vi "Get-pulse-durations.vi"(8 "error in (no error)":errorcluster) -> (0 "error out":errorcluster, 2 "Formatted contents":string)   [LabVIEW 2013, in "MaterialCharacterization.lvlib" / "MC-SM1000.lvclass"]
uses:
  MC-SM1000.lvclass
panel:
  in  "Raw signal":u8[](array[numeric])
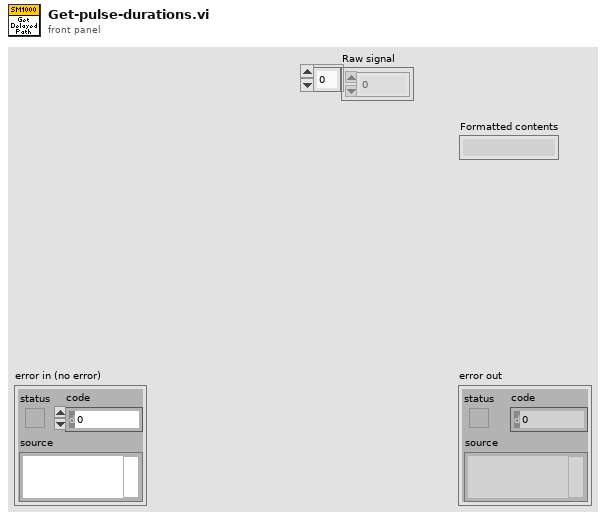
[diagram p1: front panel]
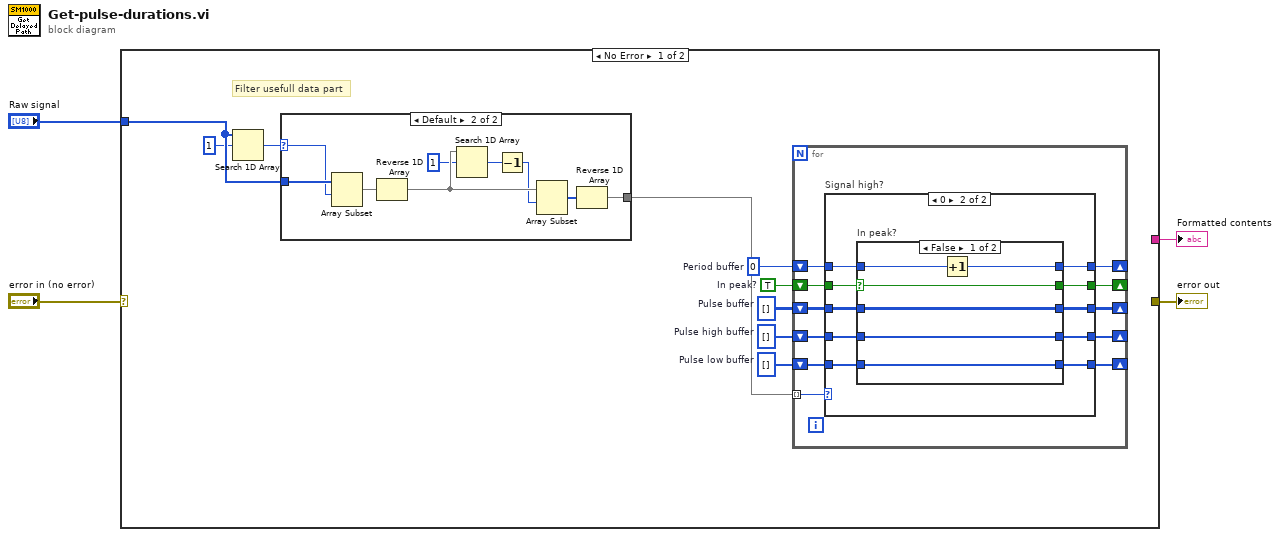
[diagram p0: block diagram]
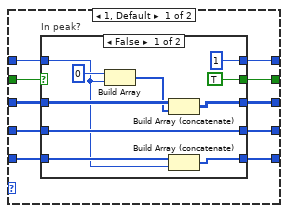
[diagram p2: hidden frame]
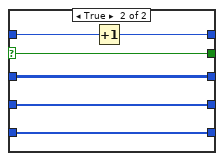
[diagram p3: hidden frame]
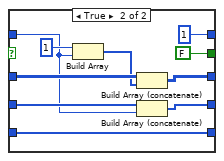
[diagram p4: hidden frame]
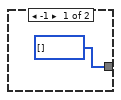
[diagram p5: hidden frame]
diagram:
  n1 = case shown="No Error" "error in (no error)" {
    selector: "error in (no error)" -> [_ w87]
    tunnel: [_ w87] -> w3
    tunnel: "Raw signal" -> [w12 _]
    tunnel: [_ _] -> w2
    frame No Error {
      w6 = i32[] []  # Pulse low buffer
      w7 = i32[] []  # Pulse high buffer
      w8 = i32[][] []  # Pulse buffer
      w9 = 0  # Period buffer
      w10 = TRUE  # In peak?
      # "Filter usefull data part"
      n2 = Search 1D Array(1D array=w12, element=u8 1) -> (index of element=w13:i32)  [unwired: 1 in]
      n3 = case shown="Default" w13 {
        selector: w13 -> [_ w79]
        tunnel: [u8[] [] w81] -> w5
        tunnel: w12 -> [_ w80]
        frame -1 {
        }
        frame Default {
          n4 = Array Subset(array=w80, index=w79) -> (w86:u8[])  [unwired: 1 in]
          n5 = Reverse 1D Array(array=w86) -> (reversed array=w84:u8[])
          n6 = Search 1D Array(1D array=w84, element=u8 1) -> (index of element=w85:i32)  [unwired: 1 in]
          n7 = Decrement(x=w85) -> (x-1=w82:i32)
          n8 = Array Subset(array=w84, index=w82) -> (w83:u8[])  [unwired: 1 in]
          n9 = Reverse 1D Array(array=w83) -> (reversed array=w81:u8[])
        }
      }
      n10 = for {
        tunnel: w5 -> [w18] mode=indexing
        shift-right: [w22] -> _
        shift-left: w8 -> [w23]
        shift-right: [w20] -> _
        shift-left: w9 -> [w21]
        shift-right: [w19] -> _
        shift-left: w10 -> [w24]
        shift-right: [w15] -> _
        shift-left: w7 -> [w17]
        shift-right: [w14] -> _
        shift-left: w6 -> [w16]
        n11 = case "Signal high?" shown="0" w18 {
          tunnel: w24 -> [w34 w60]
          tunnel: w23 -> [w33 w59]
          tunnel: [w32 w58] -> w22
          tunnel: w21 -> [w31 w57]
          tunnel: [w30 w56] -> w20
          tunnel: [w29 w55] -> w19
          tunnel: w17 -> [w28 w54]
          tunnel: w16 -> [w27 w52]
          tunnel: [w26 w53] -> w15
          tunnel: [w25 w51] -> w14
          frame 1, Default {
            n12 = case "In peak?" shown="False" w34 {
              selector: w34 -> [_ w48]
              tunnel: w33 -> [w42 w50]
              tunnel: [w41 w50] -> w32
              tunnel: w31 -> [w35 w49]
              tunnel: [1 w47] -> w30
              tunnel: [TRUE w48] -> w29
              tunnel: w28 -> [w38 w46]
              tunnel: w27 -> [w37 w45]
              tunnel: [w38 w46] -> w26
              tunnel: [w36 w45] -> w25
              frame False {
                n13 = Build Array(0, w35) -> (w40:i32[])
                n14 = Build Array (concatenate)(w42, w40) -> (w41:i32[][])
                n15 = Build Array (concatenate)(w37, w35) -> (w36:i32[])
              }
              frame True {
                n16 = Increment(x=w49) -> (x+1=w47:i32)
              }
            }
          }
          frame 0 {
            n17 = case "In peak?" shown="False" w60 {
              selector: w60 -> [w64 _]
              tunnel: w59 -> [w66 w74]
              tunnel: [w66 w73] -> w58
              tunnel: w57 -> [w65 w67]
              tunnel: [w63 1] -> w56
              tunnel: [w64 FALSE] -> w55
              tunnel: w54 -> [w62 w70]
              tunnel: [w62 w69] -> w53
              tunnel: w52 -> [w61 w68]
              tunnel: [w61 w68] -> w51
              frame False {
                n18 = Increment(x=w65) -> (x+1=w63:i32)
              }
              frame True {
                n19 = Build Array(1, w67) -> (w72:i32[])
                n20 = Build Array (concatenate)(w74, w72) -> (w73:i32[][])
                n21 = Build Array (concatenate)(w70, w67) -> (w69:i32[])
              }
            }
          }
        }
      }
    }
    frame Error {
    }
  }
  "error out" <- w3
  "Formatted contents" <- w2
